vi "Open Python 3.9 Session.vi"() -> (0 "error out":errorcluster, 3 "Refnum out":refnum<k35>)   [LabVIEW 2019]
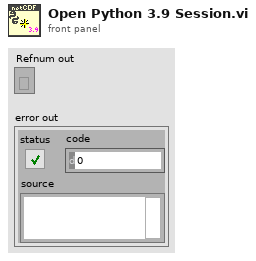
[diagram p1: front panel]
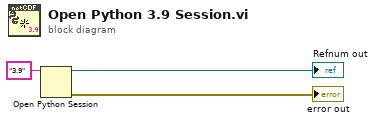
[diagram p0: block diagram]
diagram:
  n1 = Open Python Session(python version="3.9" ("Python version")) -> (session out=→"Refnum out":refnum<k35>, error out=→"error out":errorcluster)  [unwired: 2 in]
